vi "GT Get Double Var.vi"(8 "error in (no error)":errorcluster caption="错误输入（无错误）", 9 "pValue":dbl, 10 "index":i16, 11 "cardNum":i16) -> (0 "error out":errorcluster caption="错误输出", 1 "pValue out":dbl, 3 "function return":i16)   [LabVIEW 2014, in "gts.lvlib"]
doc: "GT_API GT_GetDoubleVar(short cardNum,short index,double *pValue);"
uses:
  gts.lvlib
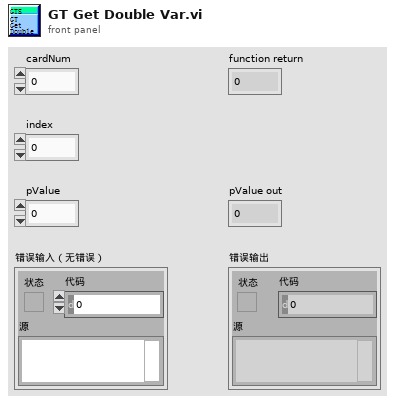
[diagram p1: front panel]
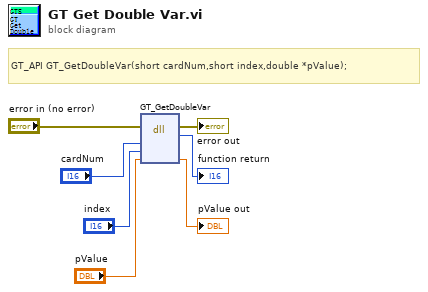
[diagram p0: block diagram]
diagram:
  # "GT_API GT_GetDoubleVar(short cardNum,short index,double *pValue);"
  n1 = dll-call lib="PTH2habs D固高科技资料GTS控制卡GTS卡18年上半年资料dllVC32bit\nmulti_cardgts.*" fn="GT_GetDoubleVar"(error in="error in (no error)", "cardNum"="cardNum", "index"="index", "pValue"="pValue") -> (error out=→"error out":errorcluster, →"function return":i16, "pValue"=→"pValue out":dbl)  [unwired: 4 in, 1 out]
